vi "Add Point.vi"(8 "error in (no error)":errorcluster, 10 "point":dbl[](array[numeric]), 11 "Locus Recorder in":refnum<class "Locus Recorder.lvclass">) -> (0 "error out":errorcluster, 3 "Locus Recorder out":refnum<class "Locus Recorder.lvclass">)   [LabVIEW 2014, in "Locus Recorder.lvclass"]
uses:
  Locus Recorder.lvclass
  Locus Recorder.lvclass/Locus Recorder.ctl
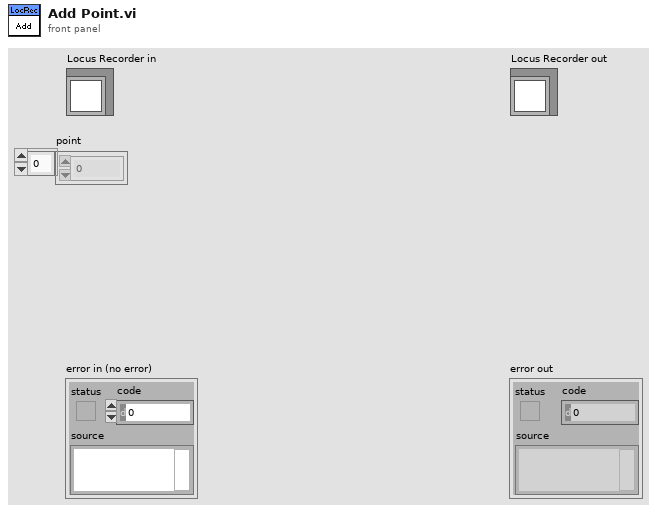
[diagram p1: front panel]
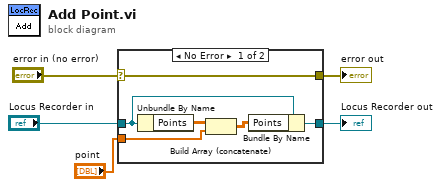
[diagram p0: block diagram]
diagram:
  n1 = case shown="No Error" "error in (no error)" {
    selector: "error in (no error)" -> [w11 w12]
    tunnel: [w11 w12] -> w4
    tunnel: [w6 w13] -> w2
    tunnel: "Locus Recorder in" -> [w8 w13]
    tunnel: "point" -> [w9 _]
    frame No Error {
      n2 = Unbundle By Name(w8) -> ("Points"=w10:dbl[][])
      n3 = Build Array (concatenate)(w10, w9) -> (w7:dbl[][])
      n4 = Bundle By Name(cluster=w8, "Points"=w7) -> (w6:refnum<class "Locus Recorder.lvclass">)
    }
    frame Error {
    }
  }
  "error out" <- w4
  "Locus Recorder out" <- w2
